vi "Create.vi"(8 "error in (no error)":errorcluster, 10 "Config Path":path) -> (0 "error out":errorcluster, 3 "System Config Module out":refnum<class "System Config Module.lvclass">)   [LabVIEW 2020, in "Volatus.lvlib" / "System Config Module.lvclass"]
uses:
  System Config Module.lvclass
  System Config Module.lvclass/System Config Module.ctl
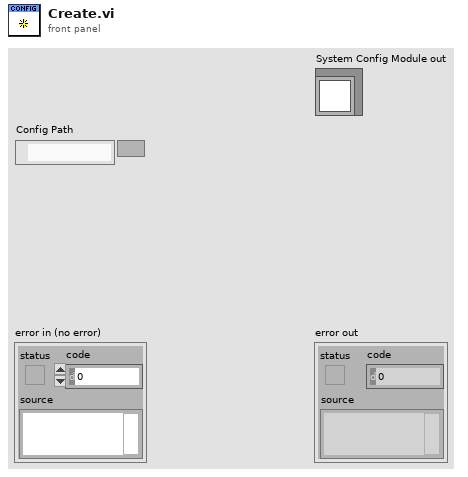
[diagram p1: front panel]
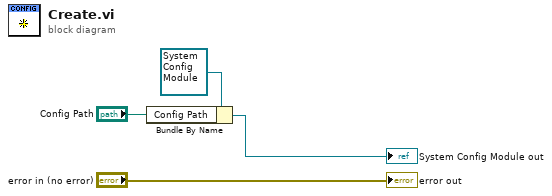
[diagram p0: block diagram]
diagram:
  n1 = Bundle By Name(cluster=refnum<class "System Config Module.lvclass"> refnum ("System Config Module in"), "Config Path"="Config Path") -> (→"System Config Module out":refnum<class "System Config Module.lvclass">)
  "error out" <- "error in (no error)"
